vi "Get Path Node VI.vi"(8 "error in (no error)":errorcluster, 11 "Node ref in":refnum<k20>) -> (0 "error out":errorcluster, 1 "Found ?":bool, 2 "VI Name out":string, 3 "Node ref out":refnum<k20>)   [LabVIEW 2020, in "LVLIBP CD XML Updater.lvlib" / "Project XML Editor.lvclass"]
uses:
  Project XML Editor.lvclass
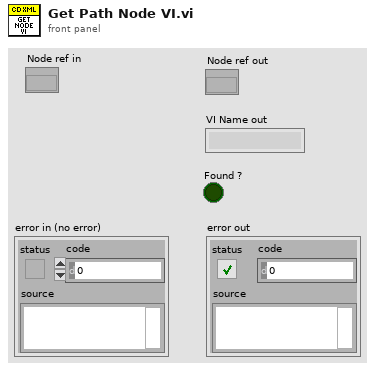
[diagram p1: front panel]
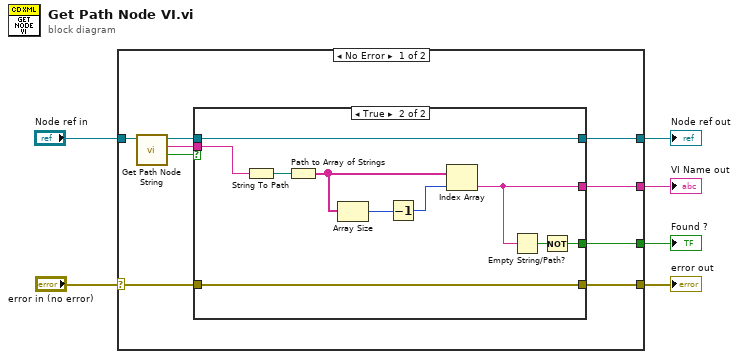
[diagram p0: block diagram]
diagram:
  n1 = case shown="No Error" "error in (no error)" {
    selector: "error in (no error)" -> [w10 w31]
    tunnel: "Node ref in" -> [w15 w30]
    tunnel: [w9 w31] -> w4
    tunnel: [w12 w30] -> w3
    tunnel: [w8 _] -> w2
    tunnel: [w7 _] -> w1
    frame No Error {
      n2 = call "Get Path Node String.vi"("Node ref in"=w15) -> ("Found ?"=w14:bool, "Path out"=w11:string, "Node ref out"=w13:refnum<k20>)  [unwired: 7 in, 1 out]
      n3 = case shown="True" w14 {
        selector: w14 -> [w16 _]
        tunnel: w11 -> [w18 w29]
        tunnel: [w18 w22] -> w7
        tunnel: w13 -> [w19 w26]
        tunnel: [w19 w26] -> w12
        tunnel: w10 -> [w17 w25]
        tunnel: [w17 w25] -> w9
        tunnel: [w16 w20] -> w8
        frame False {
        }
        frame True {
          n4 = String To Path(string=w29) -> (path=w28:path)
          n5 = Path to Array of Strings(0:w28) -> (2:w27:string[])  [unwired: 1 out]
          n6 = Array Size(array=w27) -> (size(s)=w24:i32)
          n7 = Decrement(x=w24) -> (x-1=w23:i32)
          n8 = Index Array(array=w27, index=w23) -> (element=w22:string)
          n9 = Empty String/Path?(string/path=w22) -> (empty?=w21:bool)
          n10 = Not(x=w21) -> (.not. x?=w20:bool)
        }
      }
    }
    frame Error {
    }
  }
  "VI Name out" <- w1
  "error out" <- w4
  "Node ref out" <- w3
  "Found ?" <- w2
